vi "DequeMessage.vi"(8 "error in":errorcluster, 9 "timeout in ms (-1)":i32=-1, 11 "Message que":T1) -> (0 "error out":errorcluster, 1 "Message Payload":variant, 2 "Message Command":string, 3 "Message que out":T1, 4 "Quit?":bool, 6 "timed out?":bool)   [LabVIEW 2019, in "MessageQue.lvlib"]
doc: "Receive a message.\nThis VI pulls messages off the Message Queue. \n\nBolder Software LLC"
uses:
  MessageQue.lvlib
  MessageQue.ctl
  MessageCluster.ctl
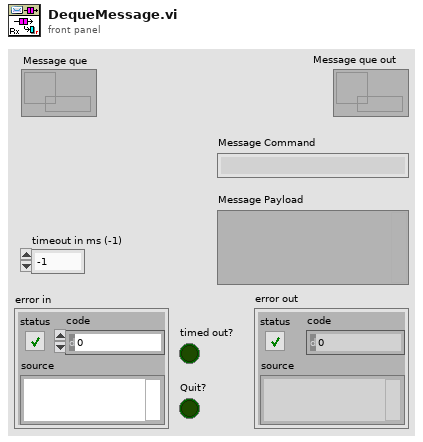
[diagram p1: front panel]
types:
  T1 = typedef "MessageQue.lvlib/MessageQue.ctl" = refnum<queue>
  T2 = typedef "MessageQue.lvlib/MessageCluster.ctl" = cluster{"Command":string, "Payload":variant}
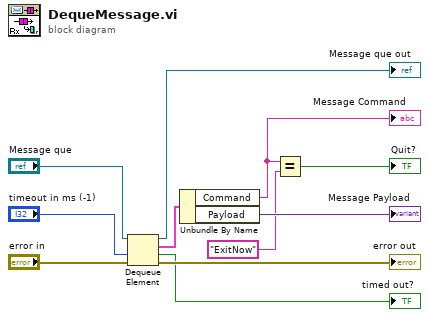
[diagram p0: block diagram]
diagram:
  n1 = Dequeue Element(queue="Message que", timeout in ms (-1)="timeout in ms (-1)", error in (no error)="error in") -> (queue out=→"Message que out":T1, element=w6:T2, timed out?=→"timed out?":bool, error out=→"error out":errorcluster)
  n2 = Unbundle By Name(w6) -> ("Command"=w2:string, "Payload"=→"Message Payload":variant)
  "Message Command" <- w2
  n3 = Equal?(x=w2, y="ExitNow") -> (x = y?=→"Quit?":bool)
